vi "enable timing reporting.vi"(8 "error in":errorcluster, 10 "timing reporting":T1, 11 "Standard Engine Configuration in":refnum<class "Standard Engine Configuration.lvclass">) -> (0 "error out":errorcluster, 3 "Standard Engine Configuration out":refnum<class "Standard Engine Configuration.lvclass">)   [LabVIEW 2013, in "Standard Engine Configuration.lvclass"]
uses:
  Standard Engine Configuration.lvclass
  timing reporting tags.ctl
  <vilib>/NI/Tag Bus/tag/Data Type.ctl
  <vilib>/NI/CEF/CEF_TreeControl/serializable configuration/NISE_CEF_serializable configuration.lvclass/NISE_CEF_serializable configuration.ctl
  <vilib>/NI/CEF/CEF_TreeControl/serializable configuration/NISE_CEF_serializable configuration.lvclass
  Standard Engine Configuration.lvclass/Standard Engine Configuration.ctl
  <vilib>/NI/Tag Bus Module Framework/channel/channel classification.ctl
  <vilib>/NI/Tag Bus/tag/tag descriptor.lvclass
  <vilib>/NI/CEF/CEF_TreeControl/serializable configuration/Read UID.vi
  <vilib>/NI/Module Execution Interface/Engine Configuration/engine configuration.lvclass
  <vilib>/NI/Tag Bus Module Framework/root configuration/TBM configuration.lvclass
  <vilib>/NI/Tag Bus Module Framework/channel/TBM channel.lvclass
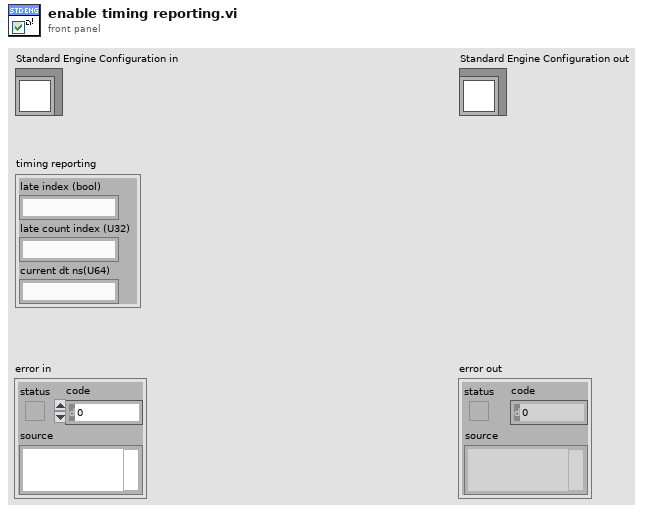
[diagram p1: front panel]
types:
  T1 = typedef "Standard Engine Configuration.lvclass/timing reporting tags.ctl" = cluster{"late index (bool)":string, "late count index (U32)":string, "current dt ns(U64)":string}
  T2 = typedef "tag bus.lvlib/tag descriptor.lvclass/Data Type.ctl" = enum16{"Double", "Single", "I64", "I32", "I16", "I8", "U64", "U32", "U16", "U8", "Boolean", "String", "Array of Double", "Array of Single", "Array of I64", "Array of I32", "Array of I16", "Array of I8", "Array of U64", "Array of U32", "Array of U16", "Array of U8", "Array of Boolean", "Array of String"}
  T3 = typedef "TBM channel.lvclass/channel classification.ctl" = enum16{"input data", "output data", "processing parameter", "processing result"}
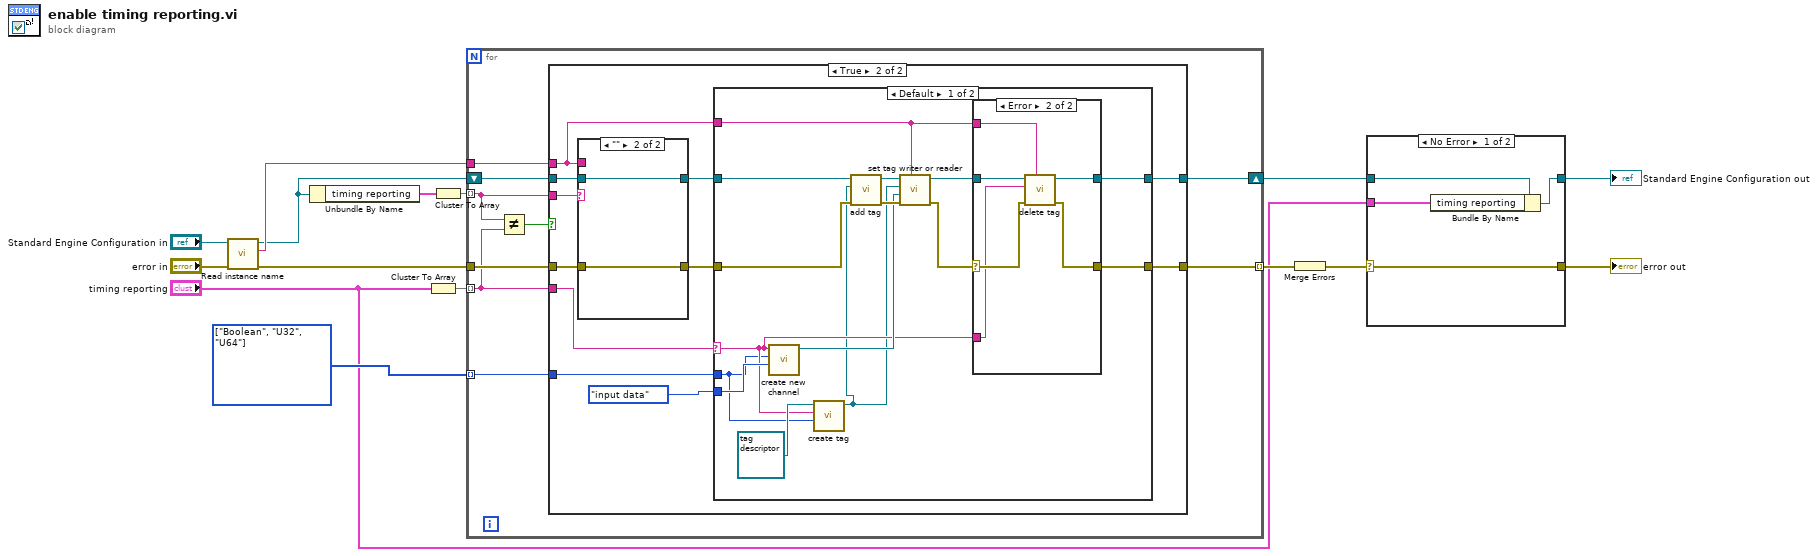
[diagram p0: block diagram]
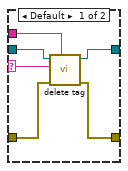
[diagram p6: hidden frame]
diagram:
  w10 = T2[] [enum."Boolean", enum."U32", enum."U64"] items=["Double", "Single", "I64", "I32", "I16", "I8", "U64", "U32", "U16", "U8", "Boolean", "String", "Array of Double", "Array of Single", "Array of I64", "Array of I32", "Array of I16", "Array of I8", "Array of U64", "Array of U32", "Array of U16", "Array of U8", "Array of Boolean", "Array of String"]
  n1 = call <vilib>:"Read instance name.vi"("error in"="error in", "configuration in"="Standard Engine Configuration in") -> ("error out"=w9:errorcluster, "instance id"=w8:string, "configuration out"=w6:refnum<class "Standard Engine Configuration.lvclass">)  [unwired: 7 in]
  n2 = Unbundle By Name(w6) -> ("timing reporting"=w13:T1)
  n3 = Cluster To Array(cluster="timing reporting") -> (array=w11:string[])
  n4 = Cluster To Array(cluster=w13) -> (array=w12:string[])
  n5 = for {
    tunnel: w12 -> [w22] mode=indexing
    tunnel: w11 -> [w17] mode=indexing
    tunnel: w10 -> [w23] mode=indexing
    shift-right: [w16] -> w5
    shift-left: w6 -> [w21]
    tunnel: w9 -> [w20]
    tunnel: [w19] -> w7 mode=indexing
    tunnel: w8 -> [w18]
    n6 = Not Equal?(x=w22, y=w17) -> (x != y?=w24:bool)
    n7 = case shown="True" w24 {
      tunnel: w23 -> [_ w31]
      tunnel: w22 -> [_ w37]
      tunnel: w21 -> [w26 w36]
      tunnel: w20 -> [w25 w35]
      tunnel: [w25 w27] -> w19
      tunnel: w18 -> [_ w29]
      tunnel: w17 -> [_ w34]
      tunnel: [w26 w28] -> w16
      frame False {
      }
      frame True {
        n8 = case shown="\"\"" w37 {
          selector: w37 -> [w68 _]
          tunnel: w36 -> [w67 w70]
          tunnel: [w66 w70] -> w33
          tunnel: w35 -> [w65 w69]
          tunnel: [w64 w69] -> w32
          tunnel: w29 -> [w63 _]
          frame Default {
            n9 = call <vilib>:"delete tag.vi"("owner ID"=w63, "error in"=w65, "tag name"=w68, "engine configuration in"=w67) -> ("error out"=w64:errorcluster, "engine configuration out"=w66:refnum<class "Standard Engine Configuration.lvclass">)  [unwired: 6 in]
          }
          frame "" {
          }
        }
        n10 = case shown="Default" w34 {
          selector: w34 -> [w40 _]
          tunnel: w33 -> [w49 w61]
          tunnel: [w45 w62] -> w27
          tunnel: w32 -> [w48 w62]
          tunnel: [w44 w61] -> w28
          tunnel: w31 -> [w39 _]
          tunnel: channel_classification."input data" ("channel classification") -> [w52 _]
          tunnel: w29 -> [w42 _]
          frame Default {
            n11 = call <vilib>:"create new channel.vi"("channel classification"=w52, "data type"=w39, "channel name"=w40) -> ("channel"=w47:refnum<class "TBM channel.lvclass">)  [unwired: 8 in]
            n12 = call-dynamic "create tag.vi"("data type"=w39, "name"=w40, "tag descriptor in"=refnum<class "tag descriptor.lvclass"> refnum) -> ("tag descriptor out"=w38:refnum<class "tag descriptor.lvclass">)  [unwired: 7 in, 1 out]
            n13 = call <vilib>:"add tag.vi"("error in"=w48, "tag descriptor"=w38, "engine configuration in"=w49) -> ("error out"=w50:errorcluster, "engine configuration out"=w51:refnum<class "Standard Engine Configuration.lvclass">)  [unwired: 7 in]
            n14 = call <vilib>:"set tag writer or reader.vi"("module GUID"=w42, "error in"=w50, "channel"=w47, "tag descriptor"=w38, "engine configuration in"=w51) -> ("error out"=w46:errorcluster, "engine configuration out"=w43:refnum<class "Standard Engine Configuration.lvclass">)  [unwired: 5 in]
            n15 = case shown="Error" w46 {
              selector: w46 -> [w54 w57]
              tunnel: [w54 w56] -> w45
              tunnel: [w53 w59] -> w44
              tunnel: w43 -> [w53 w60]
              tunnel: w42 -> [_ w58]
              tunnel: w40 -> [_ w55]
              frame No Error {
              }
              frame Error {
                n16 = call <vilib>:"delete tag.vi"("owner ID"=w58, "error in"=w57, "tag name"=w55, "engine configuration in"=w60) -> ("error out"=w56:errorcluster, "engine configuration out"=w59:refnum<class "Standard Engine Configuration.lvclass">)  [unwired: 6 in]
              }
            }
          }
          frame "" {
          }
        }
      }
    }
  }
  n17 = Merge Errors(w7) -> (w3:errorcluster)
  n18 = case shown="No Error" w3 {
    selector: w3 -> [w72 w76]
    tunnel: w5 -> [w74 w75]
    tunnel: [w73 w75] -> w4
    tunnel: [w72 w76] -> w2
    tunnel: "timing reporting" -> [w71 _]
    frame No Error {
      n19 = Bundle By Name(cluster=w74, "timing reporting"=w71) -> (w73:refnum<class "Standard Engine Configuration.lvclass">)
    }
    frame Error {
    }
  }
  "Standard Engine Configuration out" <- w4
  "error out" <- w2
